vi "AddCharacteristic.vi"(8 "error in":errorcluster, 10 "FullName":string, 11 "ProcessRun in":refnum<class "ProductUnit.lvclass">) -> (0 "error out":errorcluster, 2 "Characteristics":refnum<class "Characteristic.lvclass">, 3 "ProcessRun out":refnum<class "ProductUnit.lvclass">)   [LabVIEW 2021, in "ProligentXMLGenerator.lvlib" / "ProductUnit.lvclass"]
doc: "Add a Characteristic.\n\nA characteristic is a generic container of information that can be attached to many elements of the model.\nEach characteristic is identified by a FullName that must be unique for its owner.\nIt stores its value in a Value element.\n\nCharacteristics are unique among siblings by their FullName property.\nA characteristic is uniquely identified by the combination of its owner's identifier and its FullName"
uses:
  ProductUnit.lvclass
  ProductUnit.lvclass/ProductUnit.ctl
  Model/Characteristic/Characteristic.lvclass
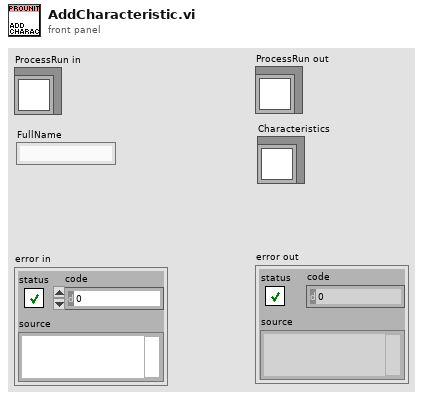
[diagram p1: front panel]
types:
  T1 = typedef "ProligentXMLGenerator.lvlib/ProductUnit.lvclass/Data.ctl" = cluster{"Name":string, "Characteristics":refnum<class "Characteristic.lvclass">[], "Documents":refnum<class "Document.lvclass">[], "CustomData":refnum<class "CustomData.lvclass">, "ProductUnitIdentifier":refnum<class "NonEmptyString_50.lvclass">, "ProductFullName":refnum<class "FullName.lvclass">, "Scrapped":refnum<class "Boolean.lvclass">, "ScrappedTime":refnum<class "DateTime.lvclass">, "CreationTime":refnum<class "DateTime.lvclass">, "ManufacturingTime":refnum<class "DateTime.lvclass">, "ByManufacturer":refnum<class "NonEmptyString_255.lvclass">, "TimeZoneInfoId":string}
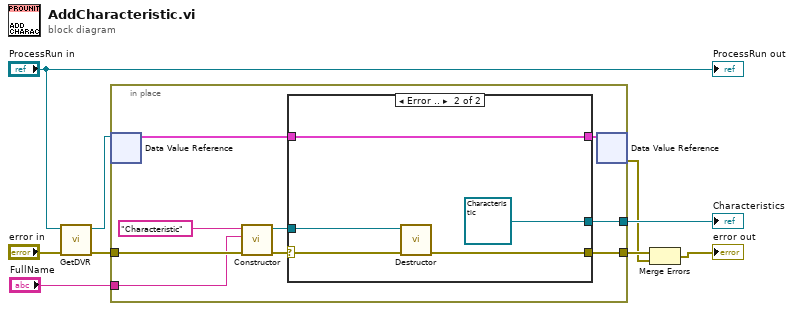
[diagram p0: block diagram]
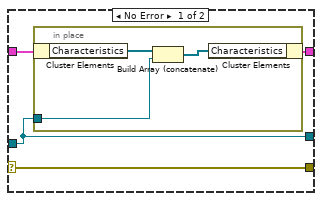
[diagram p2: hidden frame]
diagram:
  n1 = call "GetDVR.vi"("error in"="error in", "ProductUnit in"="ProcessRun in") -> ("error out"=w5:errorcluster, "DVRReference"=w4:refnum<data-value>)  [unwired: 8 in]
  n2 = in-place "In Place Element Structure" {
    in-place-border: [w18] -> w6
    in-place-border: w5 -> [w17]
    in-place-border: [w15] -> w7
    in-place-border: "FullName" -> [w11]
    n3 = in-place-dvr #1(w4) -> (w12:T1)  [unwired: 1 out]
    n4 = call "Constructor.vi"("error in"=w17, "FullName"=w11, "Name"="Characteristic") -> ("error out"=w10:errorcluster, "Document out"=w14:refnum<class "Characteristic.lvclass">)  [unwired: 7 in]
    n5 = case shown="Error .." w10 {
      selector: w10 -> [w22 w29]
      tunnel: [w19 w30] -> w16
      tunnel: [w22 w28] -> w18
      tunnel: w14 -> [w21 w27]
      tunnel: w12 -> [w20 w30]
      tunnel: [w21 refnum<class "Characteristic.lvclass"> refnum ("ProligentResultProcessor:Defect")] -> w15
      frame No Error {
        n6 = in-place "In Place Element Structure" {
          in-place-border: w21 -> [w25]
          n7 = in-place-cluster #2(w20) -> ("Characteristics"=w24:refnum<class "Characteristic.lvclass">[])
          n8 = Build Array (concatenate)(w24, w25) -> (w23:refnum<class "Characteristic.lvclass">[])
          n9 = in-place-cluster #2("Characteristics"=w23) -> (w19:T1)
        }
      }
      frame Error {
        n10 = call "Destructor.vi"("error in"=w29, "Document in"=w27) -> ("error out"=w28:errorcluster)  [unwired: 9 in]
      }
    }
    n11 = in-place-dvr #1(w16) -> (w3:errorcluster)  [unwired: 1 out]
  }
  "Characteristics" <- w7
  n12 = Merge Errors(w6, w3) -> (→"error out":errorcluster)
  "ProcessRun out" <- "ProcessRun in"
